vi "UnboxI32.vi"(10 "I32 in":refnum<class "I32.lvclass">) -> (2 "Numeric":i32)   [LabVIEW 2013, in "LapDog.Collections.v1.Common.lvlib" / "I32.lvclass"]
uses:
  I32.lvclass
  I32.lvclass/I32.ctl
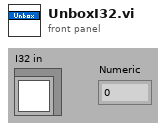
[diagram p1: front panel]
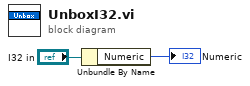
[diagram p0: block diagram]
diagram:
  n1 = Unbundle By Name("I32 in") -> ("Numeric"=→"Numeric":i32)
